vi "V to mV (DBL).vi"(8 "Boolean":bool, 11 "Input Array":dbl[](array[numeric])) -> (3 "Output Array":dbl[](array[numeric]))   [LabVIEW 2020]
doc: "Converts input signal (DBL) in volts to millivolts if Boolean input returns TRUE. Others, data flows unchanged"
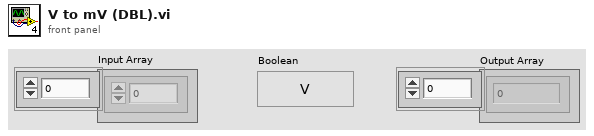
[diagram p1: front panel]
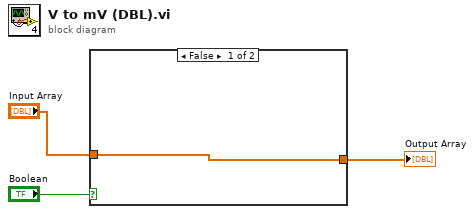
[diagram p0: block diagram]
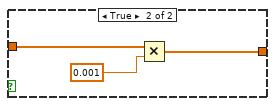
[diagram p2: hidden frame]
diagram:
  n1 = case shown="False" "Boolean" {
    tunnel: "Input Array" -> [w4 w6]
    tunnel: [w4 w5] -> w1
    frame False {
    }
    frame True {
      n2 = Multiply(x=w6, y=0.001) -> (x*y=w5:dbl[])
    }
  }
  "Output Array" <- w1
